vi "Újraolvasás.vi"(6 "Módosítás láthatóság":refnum<vi>, 9 "HIBA láthatóság":refnum<vi>, 10 "B csapat tagjai":refnum<vi>, 11 "A csapat tagjai":refnum<vi>) -> (1 "B csapat tagjai kimenet":string[](array[string]), 2 "A csapat tagjai kimenet":string[](array[string]), 3 "Mindenkinek van párja?":bool, 5 "Original file":string[][](array[string]))   [LabVIEW 2014]
doc: "Beolvassa újra, a lehetõleg már kijavított fájlt."
uses:
  <vilib>/Utility/file.llb/Read From Spreadsheet File (string).vi
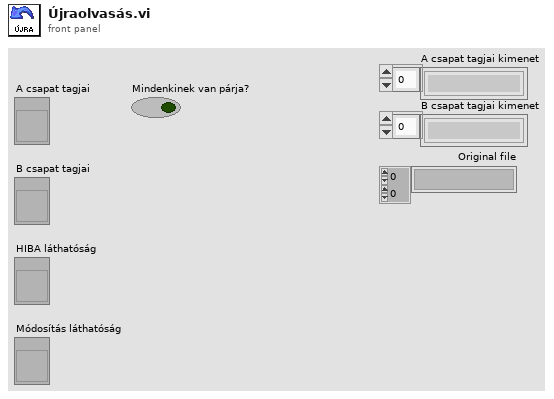
[diagram p1: front panel]
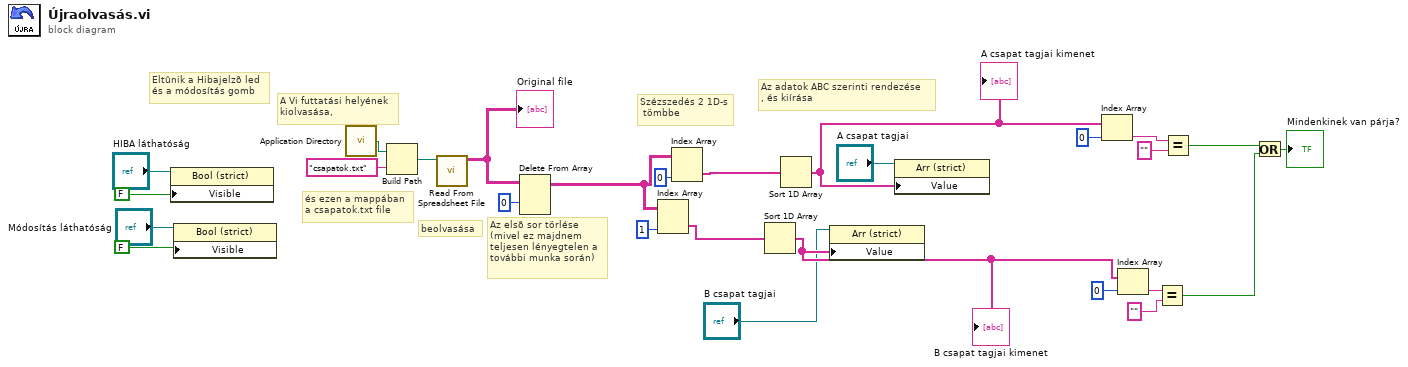
[diagram p0: block diagram]
diagram:
  # "Eltûnik a Hibajelzõ led\nés a módosítás gomb"
  # "Az elsõ sor törlése\n(mivel ez majdnem\nteljesen lényegtelen a \ntovábbi munka során)"
  # "beolvasása"
  # "és ezen a mappában\na csapatok.txt file"
  # "A Vi futtatási helyének\nkiolvasása,"
  # "Szézszedés 2 1D-s\n tömbbe"
  # "Az adatok ABC szerinti rendezése\n, és kiírása"
  n1 = property on="Property Node" class="Bool (strict)"(reference="HIBA láthatóság", "Visible"=FALSE) -> ()  [unwired: 1 in, 2 out]
  n2 = property on="Property Node" class="Bool (strict)"(reference="Módosítás láthatóság", "Visible"=FALSE) -> ()  [unwired: 1 in, 2 out]
  n3 = call <vilib>:"Application Directory.vi"() -> ("Application Directory"=w9:path)
  n4 = Build Path(base path=w9, name or relative path="csapatok.txt") -> (appended path=w14:path)
  n5 = call-poly <vilib>:"Read From Spreadsheet File.vi"("file path (dialog if empty)"=w14) -> ("all rows"=w13:string[][])  [unwired: 6 in, 4 out]
  "Original file" <- w13
  n6 = Delete From Array(array=w13, index (row)=0) -> (array with subset deleted=w12:string[][])  [unwired: 2 in, 1 out]
  n7 = Index Array(array=w12, index (col)=1 ("disabled index (col)")) -> (element=w5:string[])  [unwired: 1 in]
  n8 = Index Array(array=w12, index (col)=0 ("disabled index (col)")) -> (element=w6:string[])  [unwired: 1 in]
  n9 = Sort 1D Array(array=w5) -> (sorted array=w17:string[])
  "B csapat tagjai kimenet" <- w17
  n10 = Sort 1D Array(array=w6) -> (sorted array=w16:string[])
  "A csapat tagjai kimenet" <- w16
  n11 = property class="Arr (strict)"(reference="B csapat tagjai", "Value"=w17) -> ()  [unwired: 1 in, 2 out]
  n12 = property class="Arr (strict)"(reference="A csapat tagjai", "Value"=w16) -> ()  [unwired: 1 in, 2 out]
  n13 = Index Array(array=w16, index=0) -> (element=w23:string)
  n14 = Index Array(array=w17, index=0) -> (element=w22:string)
  n15 = Equal?(x=w22, y="") -> (x = y?=w25:bool)
  n16 = Equal?(x=w23, y="") -> (x = y?=w20:bool)
  n17 = Or(x=w20, y=w25) -> (x .or. y?=→"Mindenkinek van párja?":bool)
